vi "区间重采样.vi"(6 "时间清零":bool, 8 "重采样间隔":dbl, 9 "最小值":dbl, 10 "最大值":dbl, 11 "输出簇":cluster{"时间":dbl[], "力":dbl[]}) -> (3 "簇":cluster{"xi used":dbl[], "yi":dbl[]})   [LabVIEW 2015]
uses:
  <vilib>/gmath/NI_Gmath.lvlib
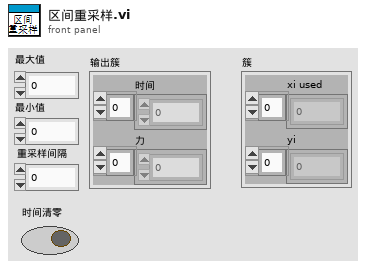
[diagram p1: front panel]
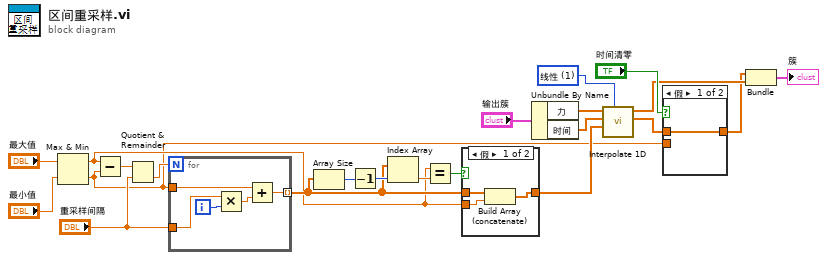
[diagram p0: block diagram]
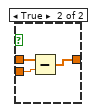
[diagram p2: hidden frame]
diagram:
  w15 = 1 items=["最近", "线性", "样条", "cubic Hermite", "拉格朗日"] ("method")
  n1 = Max & Min(x="最大值", y="最小值") -> (max(x,y)=w6:dbl, min(x,y)=w5:dbl)
  n2 = Subtract(x=w6, y=w5) -> (x-y=w22:dbl)
  n3 = Quotient & Remainder(x=w22, y="重采样间隔") -> (floor(x/y)=w20:dbl)  [unwired: 1 out]
  n4 = for {
    N: w20 -> [_]
    tunnel: "重采样间隔" -> [w26]
    tunnel: w5 -> [w24]
    tunnel: [w23] -> w10 mode=indexing
    i -> [w27]
    n5 = Multiply(x=w26, y=w27) -> (x*y=w25:dbl)
    n6 = Add(x=w24, y=w25) -> (x+y=w23:dbl)
  }
  n7 = Array Size(array=w10) -> (size(s)=w13:i32)
  n8 = Decrement(x=w13) -> (x-1=w14:i32)
  n9 = Index Array(array=w10, index=w14) -> (element=w12:dbl)
  n10 = Equal?(x=w6, y=w12) -> (x = y?=w11:bool)
  n11 = case shown="假" w11 {
    tunnel: w10 -> [w30 w31]
    tunnel: w6 -> [w29 _]
    tunnel: [w28 w31] -> w9
    frame False {
      n12 = Build Array (concatenate)(w30, w29) -> (w28:dbl[])
    }
    frame True {
    }
  }
  n13 = Unbundle By Name("输出簇") -> ("力"=w16:dbl[], "时间"=w17:dbl[])
  n14 = call <vilib>:"Interpolate 1D.vi"("method"=w15, "xi"=w9, "X"=w17, "Y"=w16) -> ("xi used"=w2:dbl[], "yi"=w3:dbl[])  [unwired: 5 in, 1 out]
  n15 = case shown="假" "时间清零" {
    tunnel: [w32 w35] -> w1
    tunnel: w5 -> [_ w34]
    tunnel: w2 -> [w32 w33]
    frame False {
    }
    frame True {
      n16 = Subtract(x=w33, y=w34) -> (x-y=w35:dbl[])
    }
  }
  n17 = Bundle("xi used"=w1, "yi"=w3) -> (→"簇":cluster{"xi used":dbl[], "yi":dbl[]})  [unwired: 1 in]
